vi "Check VI License Status 2011.vi"(8 "error in (no error)":errorcluster, 11 "Open VI References":refnum<vi>[](array[refnum])) -> (0 "error out":errorcluster, 3 "Non Activated VI Refs":bool[](array[boolean]))   [LabVIEW 2011]
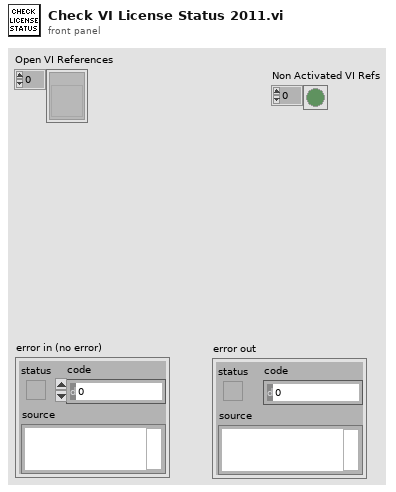
[diagram p1: front panel]
types:
  T1 = enum32{"Failure", "Activated Success", "Demo Success", "Full Demo Success"}
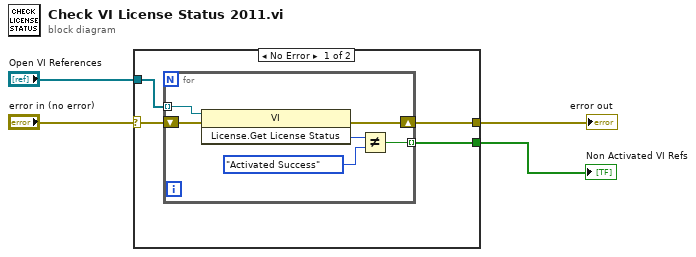
[diagram p0: block diagram]
diagram:
  n1 = case shown="No Error" "error in (no error)" {
    selector: "error in (no error)" -> [w6 w15]
    tunnel: [w8 w15] -> w4
    tunnel: "Open VI References" -> [w7 _]
    tunnel: [w5 _] -> w1
    frame No Error {
      n2 = for {
        tunnel: w7 -> [w14] mode=indexing
        tunnel: [w11] -> w5 mode=indexing
        shift-right: [w10] -> w8
        shift-left: w6 -> [w9]
        n3 = invoke class="VI" method="License.Get License Status"(reference=w14, error in=w9) -> (error out=w10:errorcluster, "License.Get License Status"=w13:T1)  [unwired: 1 in, 1 out]
        n4 = Not Equal?(x=w13, y=T1."Activated Success") -> (x != y?=w11:bool)
      }
    }
    frame Error {
    }
  }
  "error out" <- w4
  "Non Activated VI Refs" <- w1
